vi "执行系统命令.vi"() -> ()   [LabVIEW 2018]
panel:
  out "standard output":string caption="标准输出"
  out "error out":errorcluster caption="错误输出"
  in  "working directory":path=path "C:/Users/86136/Desktop/updata_data process" caption="工作目录"
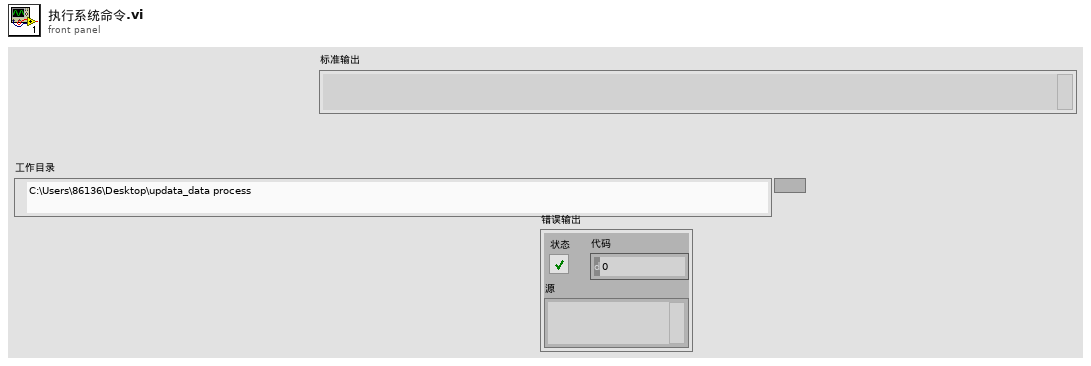
[diagram p1: front panel]
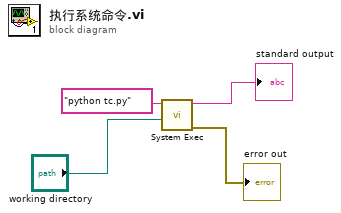
[diagram p0: block diagram]
diagram:
  n1 = call <vilib>:"System Exec.vi"("working directory"="working directory", "command line"="python tc.py") -> ("error out"=→"error out":errorcluster, "standard output"=→"standard output":string)  [unwired: 6 in, 2 out]
